vi "Calc CRC-16.vi"(3 "Frame in":u8[](array[numeric]) format="%.0x") -> (1 "CRC-16":u8[](array[numeric]) format="%.0x")   [LabVIEW 2023, in "Jiaxin_Stepper_Controller.lvlib" / "MB Master.lvlib" / "MB_ADU_RTU.lvclass"]
doc: "Calculates the 16-bit CRC of a Modbus RTU ADU (<Address><Function Code><[Data]>)"
uses:
  MB_ADU_RTU.lvclass
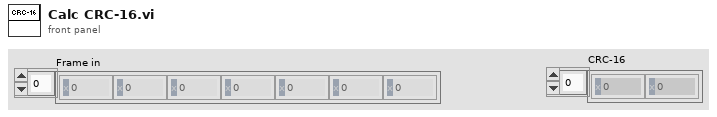
[diagram p1: front panel]
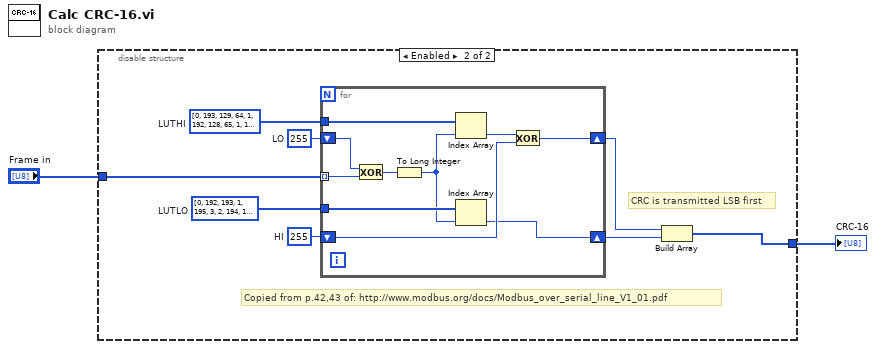
[diagram p0: block diagram]
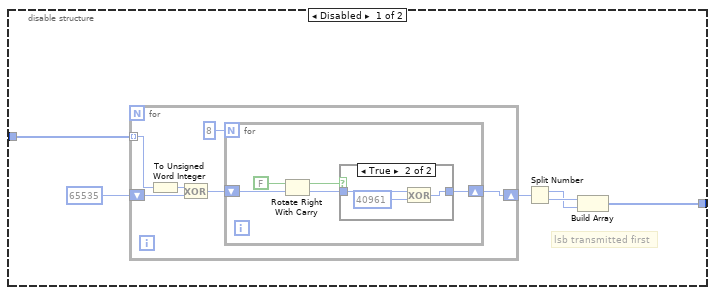
[diagram p2: hidden frame]
diagram:
  n1 = disable-structure shown="Enabled" {
    disable-tunnel: "Frame in" -> [w7 w25]
    disable-tunnel: [w3 w24] -> w1
    frame Disabled {
      # "lsb transmitted first"
      n2 = for {
        tunnel: w7 -> [w13] mode=indexing
        shift-right: [w9] -> w6
        shift-left: u16 65535 -> [w14]
        n3 = To Unsigned Word Integer(number=w13) -> (unsigned 16bit integer=w12:u16)
        n4 = Exclusive Or(1:w14, 2:w12) -> (0:w10:u16)
        n5 = for {
          N: 8 -> [_]
          shift-right: [w15] -> w9
          shift-left: w10 -> [w18]
          n6 = Rotate Right With Carry(2:w18, 3:FALSE ("carry")) -> (0:w16:u16, 1:w17:bool)
          n7 = case shown="True" w17 {
            tunnel: [w20 w21] -> w15
            tunnel: w16 -> [w20 w22]
            frame False {
            }
            frame True {
              n8 = Exclusive Or(1:u16 40961, 2:w22) -> (0:w21:u16)
            }
          }
        }
      }
      n9 = Split Number(x=w6) -> (hi(x)=w4:u8, lo(x)=w5:u8)
      n10 = Build Array(w5, w4) -> (w3:u8[])
    }
    frame Enabled {
      w29 = u8 255  # HI
      w31 = u8 255  # LO
      w28 = u8[] [0, 192, 193, 1, 195, 3, 2, 194, 198, 6, 7, 199, 5, 197, 196, 4, 204, 12, 13, 205, 15, 207, 206, 14, 10, 202, 203, 11, 201, 9, 8, 200, 216, 24, 25, 217, 27, 219, 218, 26, 30, 222, 223, 31, 221, 29, 28, 220, 20, 212, 213, 21, 215, 23, 22, 214, 210, 18, 19, 211, 17, 209, 208, 16, 240, 48, 49, 241, 51, 243, 242, 50, 54, 246, 247, 55, 245, 53, 52, 244, 60, 252, 253, 61, 255, 63, 62, 254, 250, 58, 59, 251, 57, 249, 248, 56, 40, 232, 233, 41, 235, 43, 42, 234, 238, 46, 47, 239, 45, 237, 236, 44, 228, 36, 37, 229, 39, 231, 230, 38, 34, 226, 227, 35, 225, 33, 32, 224, 160, 96, 97, 161, 99, 163, 162, 98, 102, 166, 167, 103, 165, 101, 100, 164, 108, 172, 173, 109, 175, 111, 110, 174, 170, 106, 107, 171, 105, 169, 168, 104, 120, 184, 185, 121, 187, 123, 122, 186, 190, 126, 127, 191, 125, 189, 188, 124, 180, 116, 117, 181, 119, 183, 182, 118, 114, 178, 179, 115, 177, 113, 112, 176, 80, 144, 145, 81, 147, 83, 82, 146, 150, 86, 87, 151, 85, 149, 148, 84, 156, 92, 93, 157, 95, 159, 158, 94, 90, 154, 155, 91, 153, 89, 88, 152, 136, 72, 73, 137, 75, 139, 138, 74, 78, 142, 143, 79, 141, 77, 76, 140, 68, 132, 133, 69, 135, 71, 70, 134, 130, 66, 67, 131, 65, 129, 128, 64]  # LUTLO
      w30 = u8[] [0, 193, 129, 64, 1, 192, 128, 65, 1, 192, 128, 65, 0, 193, 129, 64, 1, 192, 128, 65, 0, 193, 129, 64, 0, 193, 129, 64, 1, 192, 128, 65, 1, 192, 128, 65, 0, 193, 129, 64, 0, 193, 129, 64, 1, 192, 128, 65, 0, 193, 129, 64, 1, 192, 128, 65, 1, 192, 128, 65, 0, 193, 129, 64, 1, 192, 128, 65, 0, 193, 129, 64, 0, 193, 129, 64, 1, 192, 128, 65, 0, 193, 129, 64, 1, 192, 128, 65, 1, 192, 128, 65, 0, 193, 129, 64, 0, 193, 129, 64, 1, 192, 128, 65, 1, 192, 128, 65, 0, 193, 129, 64, 1, 192, 128, 65, 0, 193, 129, 64, 0, 193, 129, 64, 1, 192, 128, 65, 1, 192, 128, 65, 0, 193, 129, 64, 0, 193, 129, 64, 1, 192, 128, 65, 0, 193, 129, 64, 1, 192, 128, 65, 1, 192, 128, 65, 0, 193, 129, 64, 0, 193, 129, 64, 1, 192, 128, 65, 1, 192, 128, 65, 0, 193, 129, 64, 1, 192, 128, 65, 0, 193, 129, 64, 0, 193, 129, 64, 1, 192, 128, 65, 0, 193, 129, 64, 1, 192, 128, 65, 1, 192, 128, 65, 0, 193, 129, 64, 1, 192, 128, 65, 0, 193, 129, 64, 0, 193, 129, 64, 1, 192, 128, 65, 1, 192, 128, 65, 0, 193, 129, 64, 0, 193, 129, 64, 1, 192, 128, 65, 0, 193, 129, 64, 1, 192, 128, 65, 1, 192, 128, 65, 0, 193, 129, 64]  # LUTHI
      # "CRC is transmitted LSB first"
      # "Copied from p.42,43 of: http://www.modbus.org/docs/Modbus_over_serial_line_V1_01.pdf"
      n11 = for {
        tunnel: w25 -> [w40] mode=indexing
        tunnel: w30 -> [w39]
        shift-right: [w36] -> w27
        shift-left: w31 -> [w41]
        tunnel: w28 -> [w35]
        shift-right: [w32] -> w26
        shift-left: w29 -> [w37]
        n12 = Exclusive Or(1:w40, 2:w41) -> (0:w34:u8)
        n13 = To Long Integer(number=w34) -> (32bit integer=w33:i32)
        n14 = Index Array(array=w39, index=w33) -> (element=w38:u8)
        n15 = Index Array(array=w35, index=w33) -> (element=w32:u8)
        n16 = Exclusive Or(1:w37, 2:w38) -> (0:w36:u8)
      }
      n17 = Build Array(w27, w26) -> (w24:u8[])
    }
  }
  "CRC-16" <- w1
